vi "Get PC MAC Addr.vi"() -> (1 "MAC Addr":string)   [LabVIEW 2015]
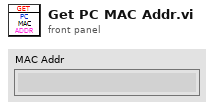
[diagram p1: front panel]
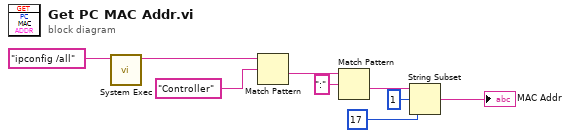
[diagram p0: block diagram]
diagram:
  n1 = call <vilib>:"System Exec.vi"("command line"="ipconfig /all") -> ("standard output"=w8:string)  [unwired: 7 in, 3 out]
  n2 = Match Pattern(string=w8, regular expression="Controller" ("Keyword")) -> (after substring=w6:string)  [unwired: 1 in, 3 out]
  n3 = Match Pattern(string=w6, regular expression=":") -> (after substring=w4:string)  [unwired: 1 in, 3 out]
  n4 = String Subset(string=w4, offset (0)=1, length (rest)=17 ("length (rest)")) -> (substring=→"MAC Addr":string)
